vi "Klinger LimitError.vi"(2 "Message d'erreur":string, 3 "Error In":errorcluster) -> (6 "Statut":bool, 8 "Error out":errorcluster)   [LabVIEW 2010]
doc: "Ce programme vérifie si l'erreur spécifié provient du controlleur (code 5001) et si elle est une fin de course (erreur 34à3B).Si oui,on efface l'erreur. Sinon, le VI \"Klinger ErrorHandler prend l'erreur en charge."
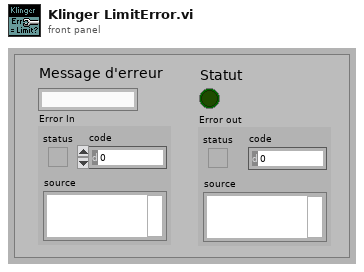
[diagram p1: front panel]
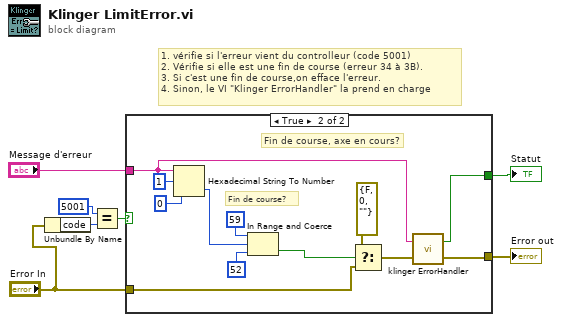
[diagram p0: block diagram]
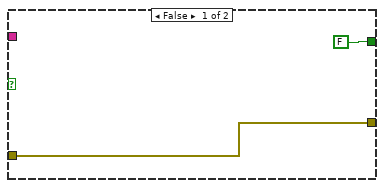
[diagram p2: hidden frame]
diagram:
  # "1. vérifie si l'erreur vient du controlleur (code 5001) \n2. Vérifie si elle est une fin de course (erreur 34 à 3B).\n3. Si c'est une fin de course,on efface l'erreur.\n4. Sinon, le VI \"Klinger ErrorHandler\" la prend en charge"
  n1 = Unbundle By Name("Error In") -> ("code"=w5:i32)
  n2 = Equal?(x=5001, y=w5) -> (x = y?=w2:bool)
  n3 = case shown="True" w2 {
    tunnel: "Message d'erreur" -> [_ w13]
    tunnel: "Error In" -> [w9 w11]
    tunnel: [w9 w12] -> w6
    tunnel: [FALSE w10] -> w1
    frame False {
    }
    frame True {
      # "Fin de course, axe en cours?"
      # "Fin de course?"
      n4 = Hexadecimal String To Number(string=w13, offset=1, default (0uL)=u8 0 ("number")) -> (number=w16:u8)  [unwired: 1 out]
      n5 = In Range and Coerce(upper limit=u8 59 ("number"), x=w16, lower limit=u8 52 ("number")) -> (In Range?=w15:bool)  [unwired: 1 out]
      n6 = Select(t=errorcluster {"status"=FALSE, "code"=0, "source"=""}, s=w15, f=w11) -> (s? t:f=w14:errorcluster)
      n7 = call <userlib>:"klinger ErrorHandler.vi"("error in (no error)"=w14, "Message D'erreur"=w13) -> ("error out"=w12:errorcluster, "Erreur"=w10:bool)
    }
  }
  "Error out" <- w6
  "Statut" <- w1
